vi "Create_String_from_JSON_Vals.vi"(11 "Model_Info_and_Report":T1={"Name"="", "Feature Extractor"="wrn_50_2_2_bnmerge", "Input3D_Custom_Dims"={"C"=0, "H"=0, "W"=0}, "Coreset Size"=0, "J-L Proj. Dim."=0, "Train_Time"=0.0, "Inf_Time"=0.0, "Feature_Layers"=[{"Layer_ID"=8, "Patch_Size"=3}, {"Layer_ID"=16, "Patch_Size"=3}], "Eval Stats(Image)"={"Scores(Good)"={"Min"=0.0, "Max"=0.0}, "Scores(Bad)"={"Min"=0.0, "Max"=0.0}, "# of Samples(Good)"=0, "# of Samples(Bad)"=0, "AUROC"=0.0, "F1_Max"=0.0, "Thrshld(F1_Max)"=0.0, "Prec.(F1_Max)"=0.0, "Recall(F1_Max)"=0.0, "FPR(F1_Max)"=0.0, "FNR(F1_Max)"=0.0}, "Eval Stats(Pixel)"={"Scores(Good)"={"Min"=0.0, "Max"=0.0}, "Scores(Bad)"={"Min"=0.0, "Max"=0.0}, "# of Samples(Good)"=0, "# of Samples(Bad)"=0, "AUROC"=0.0, "F1_Max"=0.0, "Thrshld(F1_Max)"=0.0, "Prec.(F1_Max)"=0.0, "Recall(F1_Max)"=0.0, "FPR(F1_Max)"=0.0, "FNR(F1_Max)"=0.0}} {"Eval Stats(Pixel)"."Recall(F1_Max)" format="%#.5f"; "Eval Stats(Pixel)"."FPR(F1_Max)" format="%#.5f"; "Eval Stats(Pixel)"."FNR(F1_Max)" format="%#.5f"; "Eval Stats(Pixel)"."Prec.(F1_Max)" format="%#.5f"; "Eval Stats(Pixel)"."F1_Max" format="%#.5f"; "Eval Stats(Pixel)"."AUROC" format="%#.5f"; "Eval Stats(Pixel)"."Scores(Bad)"."Min" format="%#_5g"; "Eval Stats(Pixel)"."Scores(Good)"."Min" format="%#_5g"; "Eval Stats(Pixel)"."Thrshld(F1_Max)" format="%#_5f"; "Eval Stats(Image)"."Recall(F1_Max)" format="%#.5f"; "Eval Stats(Image)"."FPR(F1_Max)" format="%#.5f"; "Eval Stats(Image)"."FNR(F1_Max)" format="%#.5f"; "Eval Stats(Image)"."Prec.(F1_Max)" format="%#.5f"; "Eval Stats(Image)"."F1_Max" format="%#.5f"; "Eval Stats(Image)"."AUROC" format="%#.5f"; "Eval Stats(Image)"."Scores(Bad)"."Min" format="%#_5g"; "Eval Stats(Image)"."Scores(Good)"."Min" format="%#_5g"; "Eval Stats(Image)"."Thrshld(F1_Max)" format="%#_5f"}) -> (3 "String":string)   [LabVIEW 2020]
uses:
  <vilib>/Ngene/Deep Learning Toolkit/Toolkit/NN_Data/API/NN_Dims(C,H,W).ctl
  <vilib>/Ngene/Deep Learning Toolkit/Toolkit/Deep_Learning_Toolkit_by_Ngene.lvlib
  HyperParam_Investigation/Controls/Model_Info_and_Report.ctl
  HyperParam_Investigation/Controls/Feature_Layers_CFG.ctl
  <vilib>/Ngene/DeepLTK Anomaly Detection Addon/DeepLTK_Anomaly_Detection_Addon/API/Controls/MinMax.ctl
  <vilib>/Ngene/DeepLTK Anomaly Detection Addon/DeepLTK_Anomaly_Detection_Addon/DeepLTK_Anomaly_Detection_Addon.lvlib
  <vilib>/Ngene/DeepLTK Anomaly Detection Addon/DeepLTK_Anomaly_Detection_Addon/API/Controls/Eval_Results.ctl
panel:
  out "number of replacements":i32
  out "result string":string
  out "spreadsheet string":string
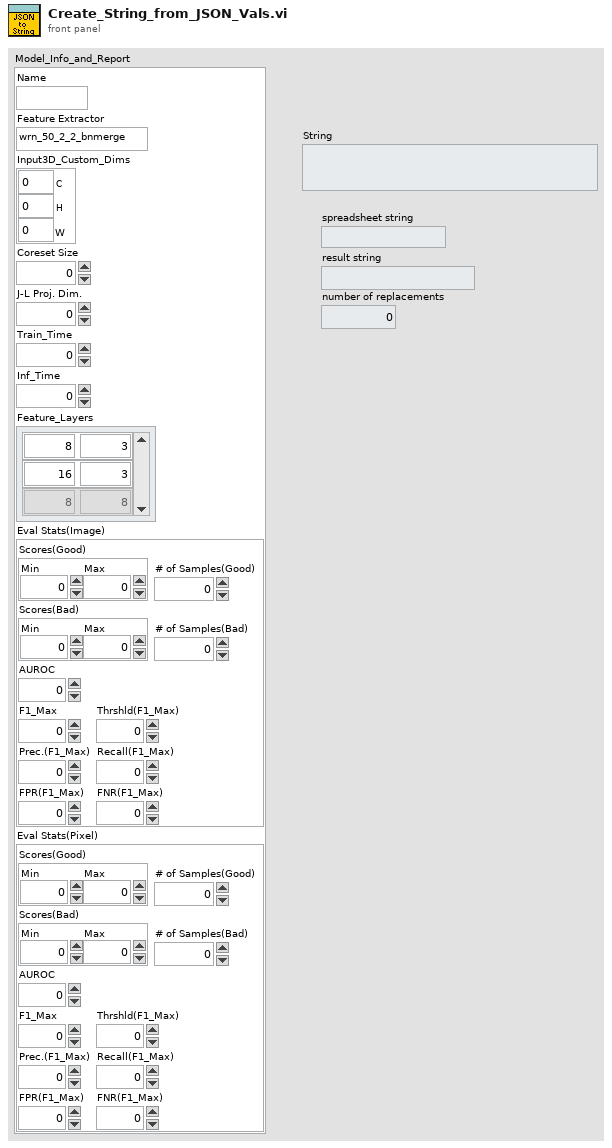
[diagram p1: front panel]
types:
  T1 = typedef "Model_Info_and_Report.ctl" = cluster{"Name":string, "Feature Extractor":string, "Input3D_Custom_Dims":T2, "Coreset Size":i32, "J-L Proj. Dim.":i32, "Train_Time":dbl, "Inf_Time":dbl, "Feature_Layers":T3, "Eval Stats(Image)":T4, "Eval Stats(Pixel)":T4}
  T2 = typedef "Deep_Learning_Toolkit_by_Ngene.lvlib/NN_Dims(C,H,W).ctl" = cluster{"C":i32, "H":i32, "W":i32}
  T3 = typedef "Feature_Layers_CFG.ctl" = cluster{"Layer_ID":i32, "Patch_Size":i32}[]
  T4 = typedef "DeepLTK_Anomaly_Detection_Addon.lvlib/Eval_Results.ctl" = cluster{"Scores(Good)":T5, "Scores(Bad)":T5, "# of Samples(Good)":i32, "# of Samples(Bad)":i32, "AUROC":sgl, "F1_Max":sgl, "Thrshld(F1_Max)":sgl, "Prec.(F1_Max)":sgl, "Recall(F1_Max)":sgl, "FPR(F1_Max)":sgl, "FNR(F1_Max)":sgl}
  T5 = typedef "DeepLTK_Anomaly_Detection_Addon.lvlib/MinMax.ctl" = cluster{"Min":sgl, "Max":sgl}
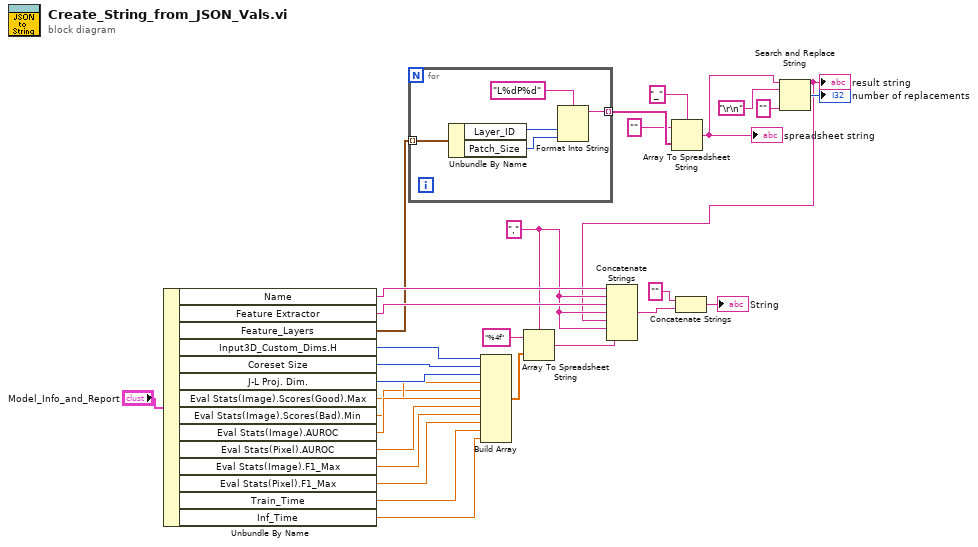
[diagram p0: block diagram]
diagram:
  w6 = "," ("delimiter (Tab)")
  n1 = Unbundle By Name("Model_Info_and_Report") -> ("Name"=w11:string, "Feature Extractor"=w12:string, "Feature_Layers"=w10:T3, "Input3D_Custom_Dims.H"=w14:i32, "Coreset Size"=w30:i32, "J-L Proj. Dim."=w17:i32, "Eval Stats(Image).Scores(Good).Max"=w16:sgl, "Eval Stats(Image).Scores(Bad).Min"=w15:sgl, "Eval Stats(Image).AUROC"=w24:sgl, "Eval Stats(Pixel).AUROC"=w25:sgl, "Eval Stats(Image).F1_Max"=w26:sgl, "Eval Stats(Pixel).F1_Max"=w27:sgl, "Train_Time"=w28:dbl, "Inf_Time"=w13:dbl)
  n2 = for {
    tunnel: w10 -> [w35] mode=indexing
    tunnel: [w31] -> w9 mode=indexing
    n3 = Unbundle By Name(w35) -> ("Layer_ID"=w34:i32, "Patch_Size"=w33:i32)
    n4 = Format Into String(format string="L%dP%d", w34, w33) -> (resulting string=w31:string)  [unwired: 2 in, 1 out]
  }
  n5 = Build Array(w14, w30, w17, w16, w15, w24, w25, w26, w27, w28, w13) -> (w29:dbl[])
  n6 = Array To Spreadsheet String(delimiter (Tab)=w6, array=w29, 3:"%4f" ("spreadsheet string")) -> (spreadsheet string=w22:string)
  n7 = Array To Spreadsheet String(delimiter (Tab)="_", array=w9, 3:"" ("format string")) -> (spreadsheet string=w2:string)
  "spreadsheet string" <- w2
  n8 = Search and Replace String(input string=w2, search string="\r\n", replace string="" ("replace string (\"\")")) -> (result string=w1:string, number of replacements=→"number of replacements":i32)  [unwired: 5 in, 2 out]
  "result string" <- w1
  n9 = Concatenate Strings(w11, w6, w12, w6, w1, w6, w22) -> (w23:string)
  n10 = Concatenate Strings("" ("spreadsheet string"), w23) -> (→"String":string)
